vi "AttitudeIndicatorMerge.vi"() -> ()   [LabVIEW 2017]
uses:
  <vilib>/robotics/Controls/Attitude Indicator/Attitude Indicator.xctl
panel:
  out "Attitude Indicator":cluster{"Roll":dbl, "Pitch":dbl}(xcontrol)
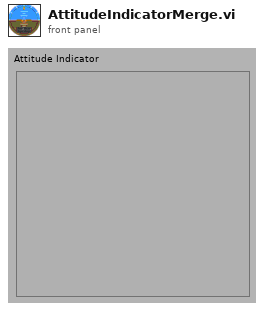
[diagram p1: front panel]
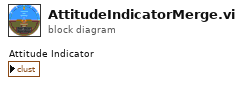
[diagram p0: block diagram]
diagram:
